vi "wait for ready.vi"(8 "error in":errorcluster, 11 "profibus reference":T1) -> (0 "error out":errorcluster, 2 "ready":bool, 3 "profibus reference out":T1)   [LabVIEW 2013, in "dynamic profibus.lvlib"]
uses:
  fpga reference.ctl
  <vilib>/rvi/interface/common/niFpgaWaitOnOcc.vi
  <vilib>/Utility/error.llb/Error Cluster From Error Code.vi
  <vilib>/rvi/errors/niLvFpgaAdjustHostInterfaceError.vi
  <vilib>/rvi/interface/nirviReadWriteControl/nirviReadWriteControl.xnode
  dynamic profibus.lvlib
  NiFpgaLv.dll
  <vilib>/rvi/interface/Simulation/niFpgaSimulationCallBeginRW.vi
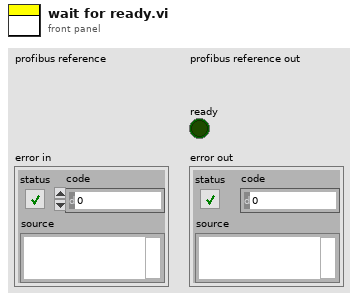
[diagram p1: front panel]
types:
  T1 = typedef "dynamic profibus.lvlib/fpga reference.ctl" = refnum<k20>
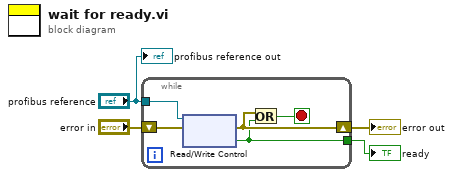
[diagram p0: block diagram]
diagram:
  n1 = while {
    tunnel: "profibus reference" -> [w9]
    shift-right: [w7] -> w2
    shift-left: "error in" -> [w8]
    tunnel: [w5] -> w1
    stop <- w6 stop-if-true
    n2 = xnode "Read/Write Control"("FPGA VI Reference In"=w9, "error in"=w8) -> ("error out"=w7:errorcluster, "ready"=w5:bool)  [unwired: 1 out]
    n3 = Or(x=w7, y=w5) -> (x .or. y?=w6:bool)
  }
  "error out" <- w2
  "ready" <- w1
  "profibus reference out" <- "profibus reference"
